vi "Replace Section Keys.vi"(7 "Section":string, 8 "error in (no error)":errorcluster, 9 "Values":string[](array[string]), 10 "Keys":string[](array[string]), 11 "INI Path":path) -> (0 "error out":errorcluster)   [LabVIEW 2017]
doc: "Writes the desired keys and values to the target section of the input INI file. If the keys use hierarchical \"dot\" notation, this VI will first delete all keys with the same hierarchy as the input keys. Use this VI if the input hierarchy includes arrays or similar complex structures. If the input keys have a flat hierarchy, use the simple Write Section Keys instead."
uses:
  <vilib>/Utility/config.llb/NI_LVConfig.lvlib
  <userlib>/Toolbox/Array Handling/Find Unique Elements/Find Unique Elements STR.vi
  <vilib>/Utility/config.llb/Write Key (String).vi
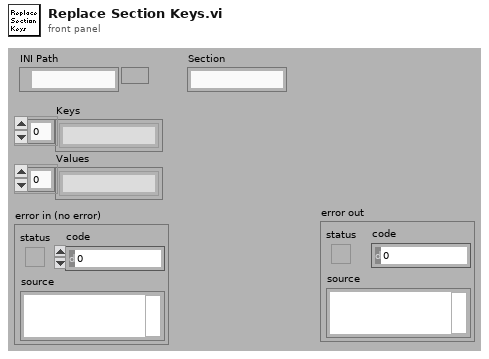
[diagram p1: front panel]
types:
  T1 = typedef "NI_LVConfig.lvlib/Config Data RefNum.ctl" = refnum<k1>
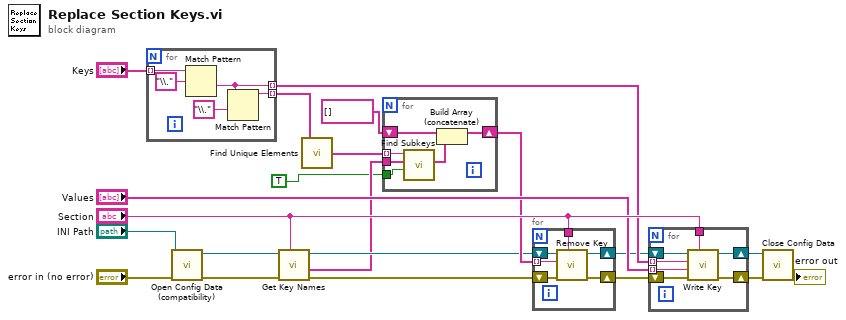
[diagram p0: block diagram]
diagram:
  n1 = for {
    tunnel: "Keys" -> [w25] mode=indexing
    tunnel: [w23] -> w2 mode=indexing
    tunnel: [w22] -> w14 mode=indexing
    n2 = Match Pattern(string=w25, regular expression="\\.") -> (after substring=w22:string)  [unwired: 1 in, 3 out]
    n3 = Match Pattern(string=w22, regular expression="\\.") -> (before substring=w23:string)  [unwired: 1 in, 3 out]
  }
  n4 = call <vilib>:"Open Config Data (compatibility).vi"("error in (no error)"="error in (no error)", "configuration file path"="INI Path") -> ("error out"=w3:errorcluster, "refnum"=w4:T1)  [unwired: 7 in, 1 out]
  n5 = call <vilib>:"Get Key Names.vi"("section"="Section", "error in (no error)"=w3, "refnum"=w4) -> ("error out"=w8:errorcluster, "key names"=w5:string[], "refnum out"=w9:T1)  [unwired: 5 in, 1 out]
  n6 = call-poly <userlib>:"Find Unique Elements.vi"("Array In"=w2) -> ("Array Out"=w6:string[])
  n7 = for {
    tunnel: w5 -> [w32]
    tunnel: w6 -> [w31] mode=indexing
    shift-right: [w30] -> w10
    shift-left: string[] [] ("Subkeys") -> [w28]
    tunnel: TRUE -> [w27]
    n8 = call "Find Subkeys.vi"("Full Path? (false)"=w27, "Keys"=w32, "Key Root"=w31) -> ("Subkeys"=w29:string[])  [unwired: 8 in]
    n9 = Build Array (concatenate)(w28, w29) -> (w30:string[])
  }
  n10 = for {
    tunnel: w10 -> [w36] mode=indexing
    shift-right: [w35] -> w12
    shift-left: w8 -> [w38]
    shift-right: [w34] -> w11
    shift-left: w9 -> [w37]
    tunnel: "Section" -> [w33]
    n11 = call <vilib>:"Remove Key.vi"("section"=w33, "error in (no error)"=w38, "key"=w36, "refnum"=w37) -> ("error out"=w35:errorcluster, "refnum out"=w34:T1)  [unwired: 5 in, 1 out]
  }
  n12 = for {
    shift-right: [w44] -> w20
    shift-left: w11 -> [w45]
    shift-right: [w42] -> w19
    shift-left: w12 -> [w43]
    tunnel: w14 -> [w41] mode=indexing
    tunnel: "Values" -> [w40] mode=indexing
    tunnel: "Section" -> [w39]
    n13 = call-poly <vilib>:"Write Key.vi"("section"=w39, "error in (no error)"=w43, "value"=w40, "key"=w41, "refnum"=w45) -> ("error out"=w42:errorcluster, "refnum out"=w44:T1)  [unwired: 4 in, 1 out]
  }
  n14 = call <vilib>:"Close Config Data.vi"("error in (no error)"=w19, "refnum"=w20) -> ("error out"=→"error out":errorcluster)  [unwired: 8 in, 1 out]
